vi "Read Wear_in.vi"(8 "error in (no error)":errorcluster, 11 "Solenoid in":refnum<class "Solenoid.lvclass">) -> (0 "error out":errorcluster, 2 "Wear_in":T1={"V"=24.0, "I"=0.5, "Cycles"=0.5, "On_Time_ms"=0.5, "Off_Time_ms"=0.5}, 3 "Solenoid out":refnum<class "Solenoid.lvclass">)   [LabVIEW 2025, in "Solenoid.lvclass"]
uses:
  Solenoid.lvclass
  Solenoid.lvclass/Solenoid.ctl
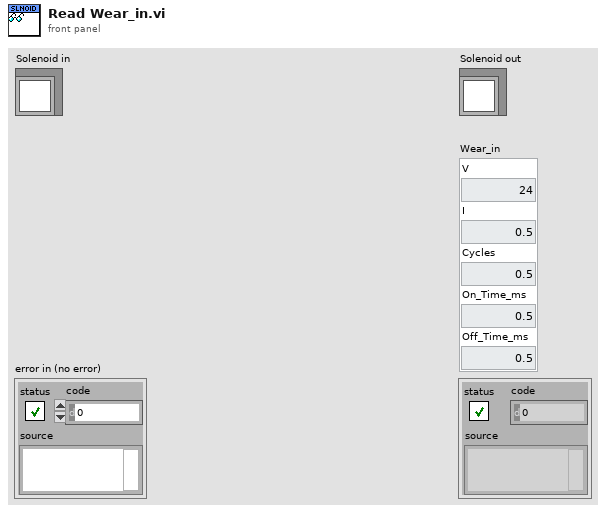
[diagram p1: front panel]
types:
  T1 = cluster{"V":dbl, "I":dbl, "Cycles":dbl, "On_Time_ms":dbl, "Off_Time_ms":dbl}
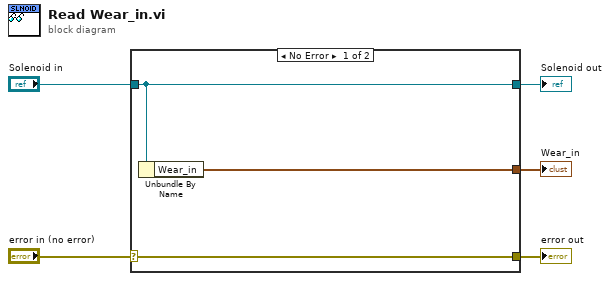
[diagram p0: block diagram]
diagram:
  n1 = case shown="No Error" "error in (no error)" {
    selector: "error in (no error)" -> [w8 w9]
    tunnel: [w8 w9] -> w4
    tunnel: [w7 w10] -> w2
    tunnel: "Solenoid in" -> [w7 w10]
    tunnel: [w6 _] -> w1
    frame No Error {
      n2 = Unbundle By Name(w7) -> ("Wear_in"=w6:T1)
    }
    frame Error {
    }
  }
  "error out" <- w4
  "Solenoid out" <- w2
  "Wear_in" <- w1
